vi "key to field and type.vi"(11 "key":u64 format="%.0x") -> (2 "wire type":T1, 3 "field number":u64)   [LabVIEW 2013, in "protocol buffers encoder.lvlib"]
uses:
  protocol buffers encoder.lvlib
  wire type.ctl
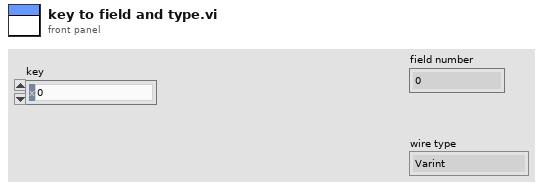
[diagram p1: front panel]
types:
  T1 = typedef "protocol buffers encoder.lvlib/wire type.ctl" = enum8{"Varint", "64 bit", "Length Delimited", "Start Group", "End Group", "32 bit"}
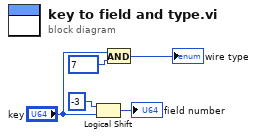
[diagram p0: block diagram]
diagram:
  n1 = Logical Shift(y=i16 -3, x="key") -> (x << y=→"field number":u64)
  n2 = And(x="key", y=u64 7) -> (x .and. y?=→"wire type":u64)
